vi "氨氮总磷质控流程.vi"(0 "队列输入":refnum<queue>, 5 "氨氮":bool, 7 "氨氮量程切换":enum32{"H", "L", "AUTO"}(ring)=enum."AUTO", 9 "总磷":bool, 11 "总磷量程切换":enum32{"H", "L", "AUTO"}(ring)=enum."AUTO") -> (4 "布尔":bool, 6 "总磷中断报警":bool, 8 "氨氮中断报警":bool)   [LabVIEW 2016, in "质控单元.lvlib"]
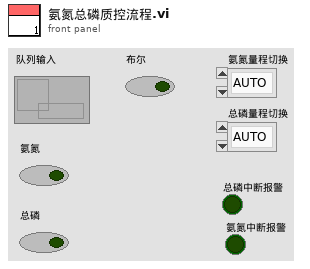
[diagram p1: front panel]
types:
  T1 = enum16{"待机", "启动氨氮水样", "氨氮测量中", "启动氨氮加标", "启动氨氮加标回收", "氨氮加标回收测量中", "启动总磷水样", "总磷水样测量中", "启动总磷加标", "启动总磷加标回收", "总磷加标回收测量中", "结束"}
  T2 = cluster{"站号":u16, "量程切换":enum32{"H", "L", "AUTO"}, "控制命令":enum16{"启动测量", "标样核查", "零点核查", "跨度核查", "空白测试", "平行样测试", "加标回收", "空白校准", "标样校准", "初始化（清洗）", "停止测试", "仪器重启", "校时", "模式设置", "测量间隔设置", "盲样测试"}, "模式设置":enum16{"待机", "连续模式", "周期模式", "定点模式", "受控模式", "手动模式"}, "测量间隔":u16}
  T3 = cluster{"时间标识":timestamp, "设备":string, "日志信息":string}
  T4 = cluster{"系统时间":timestamp, "工作状态":enum16{"空闲", "水样测试", "标样核查", "零点核查", "跨度核查", "空白测试", "平行样测试", "加标回收", "空白校准", "标样校准", "初始化（清洗）"}, "测量模式":enum16{"待机", "连续模式", "周期模式", "定点模式", "受控模式", "手动模式"}, "告警代码":enum16{"无告警", "缺试剂告警", "缺水样告警", "缺蒸馏水告警", "缺标液告警", "仪表漏液告警", "标定异常告警", "超量程告警", "加热异常", "低试剂预警", "超上限告警", "超下限告警", "仪表内部其他异常", "滴定异常告警", "电极异常告警", "量程切换告警", "参数设置告警", "PH电极电位异常", "电导率电极异常", "浊度光度异常", "溶解氧电极异常", "溶解氧光强异常", "温度异常告警", "PH异常告警", "溶解氧异常告警", "电导率异常告警", "浊度异常告警", "叶绿素异常告警", "藻密度异常告警", "蓝绿藻异常告警", "ORP异常告警", "氨氮异常告警", "清洁刷异常告警", "SD卡异常告警", "蓝牙异常告警", "Wifi异常告警", "流程异常告警"}, "故障代码":enum16{"无故障", "电机故障", "温度故障", "通讯故障", "滴定故障"}, "日志代码":u16, "软件版本":u16, "F0":sgl, "F1":sgl, "F2":sgl, "F3":sgl, "T":sgl, "H":sgl, "id":u16, "flowid":u16, "量程":u16, "总磷控温温度1":sgl, "营养盐控温温度2":sgl, "ADC":sgl}
  T5 = enum16{"空闲", "水样测试", "标样核查", "零点核查", "跨度核查", "空白测试", "平行样测试", "加标回收", "空白校准", "标样校准", "初始化（清洗）"}
  T6 = cluster{"因子编码":u32, "单位":u16, "标样参考值":sgl, "水样数据时间":timestamp, "水样实测值":sgl, "水样数据标识":string, "标样数据时间":timestamp, "标样实测值":sgl, "标样数据标识":string, "空白数据时间":timestamp, "空白实测值":sgl, "空白数据标识":string, "零点核查数据时间":timestamp, "零点核查实测值":sgl, "零点核查数据标识":string, "跨度核查数据时间":timestamp, "跨度核查实测值":sgl, "跨度核查数据标识":string, "加标回收数据时间":timestamp, "加标回收实测值":sgl, "加标回收数据标识":string, "平行样数据时间":timestamp, "平行样实测值":sgl, "平行样数据标识":string}
  T7 = cluster{"量程":dbl, "检出限":dbl, "加标前水样浓度":dbl, "加标后水样浓度":dbl, "加标水杯定容体积":dbl, "加标母液浓度":dbl, "加标体积":dbl, "加标回收率":dbl}
  T8 = cluster{"氨氮":u8, "总磷":u8, "总氮":u8, "CODMn":u8, "CODCr":u8}
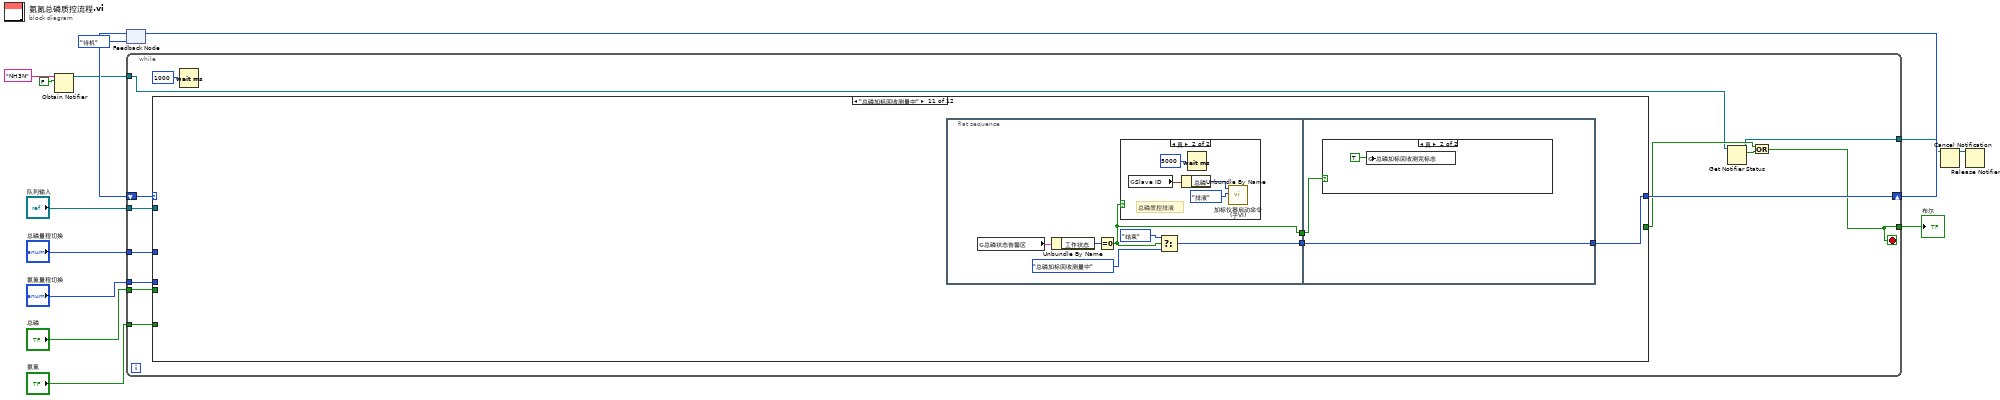
[diagram p0: block diagram]
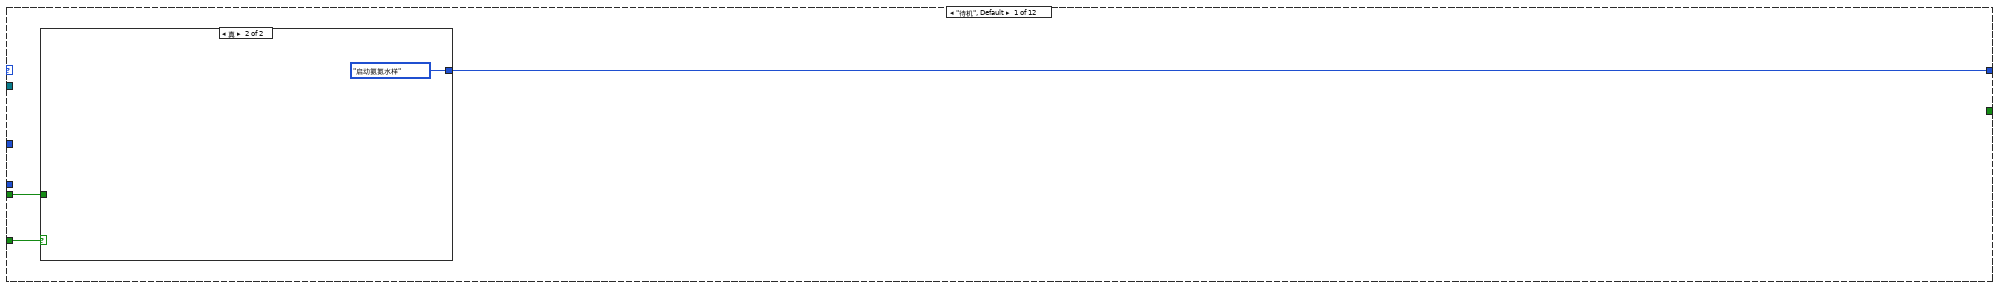
[diagram p2: hidden frame]
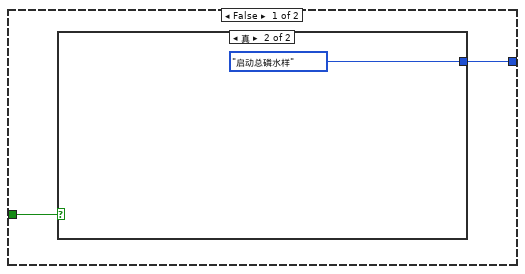
[diagram p3: hidden frame]
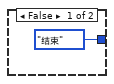
[diagram p4: hidden frame]
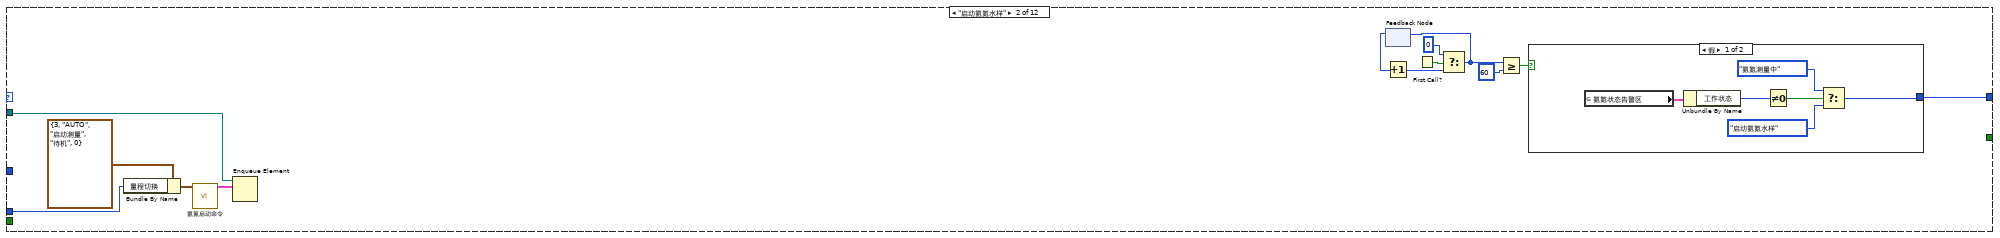
[diagram p5: hidden frame]
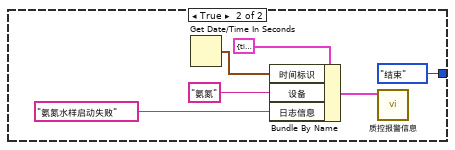
[diagram p6: hidden frame]
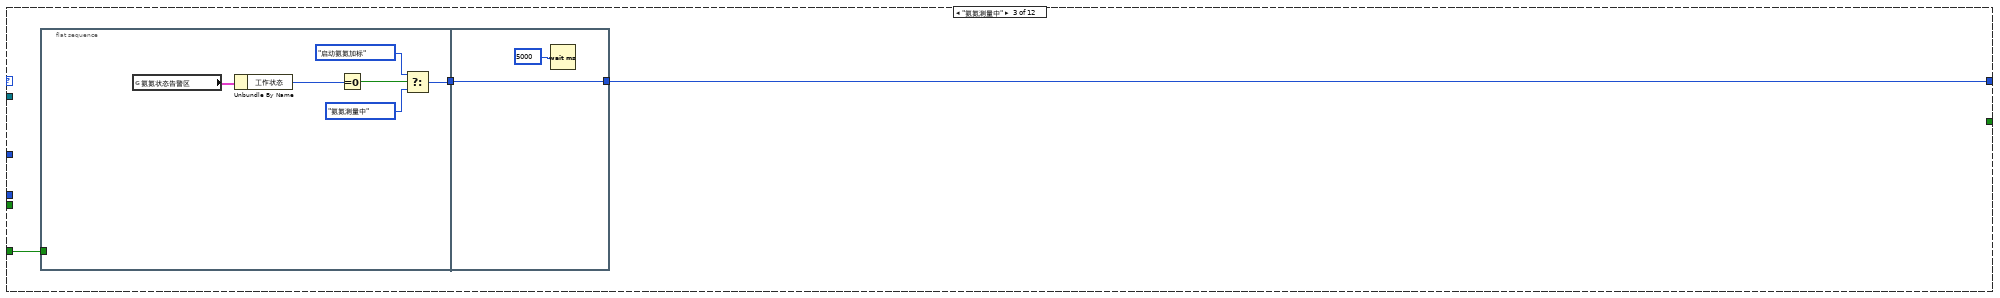
[diagram p7: hidden frame]
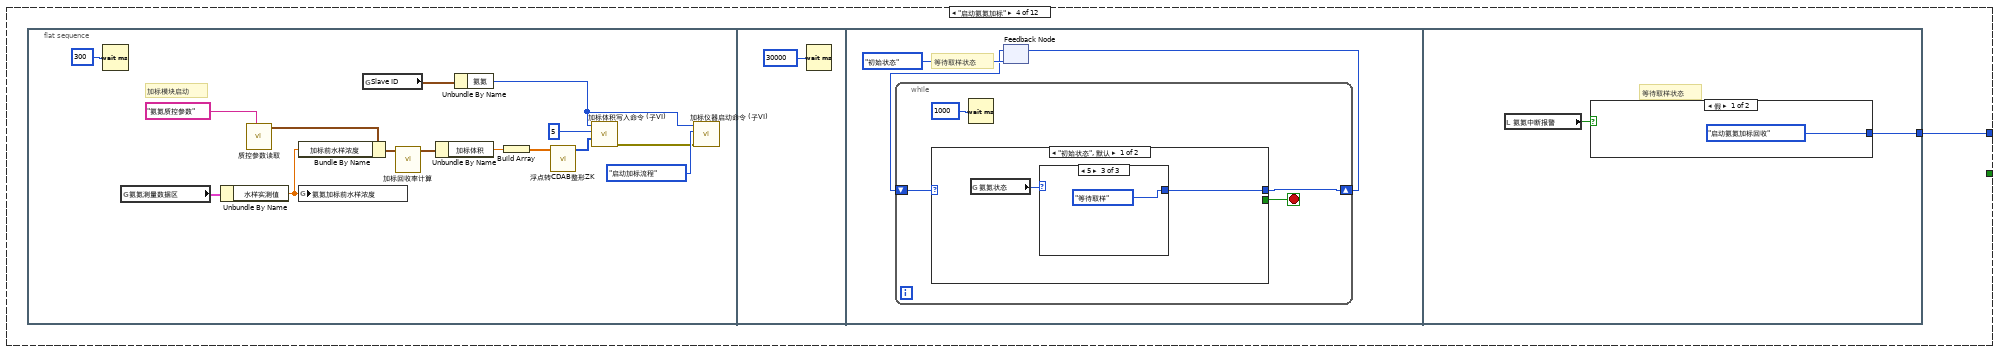
[diagram p8: hidden frame]
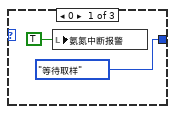
[diagram p9: hidden frame]
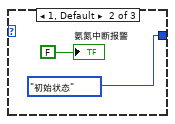
[diagram p10: hidden frame]
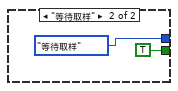
[diagram p11: hidden frame]
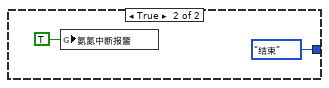
[diagram p12: hidden frame]
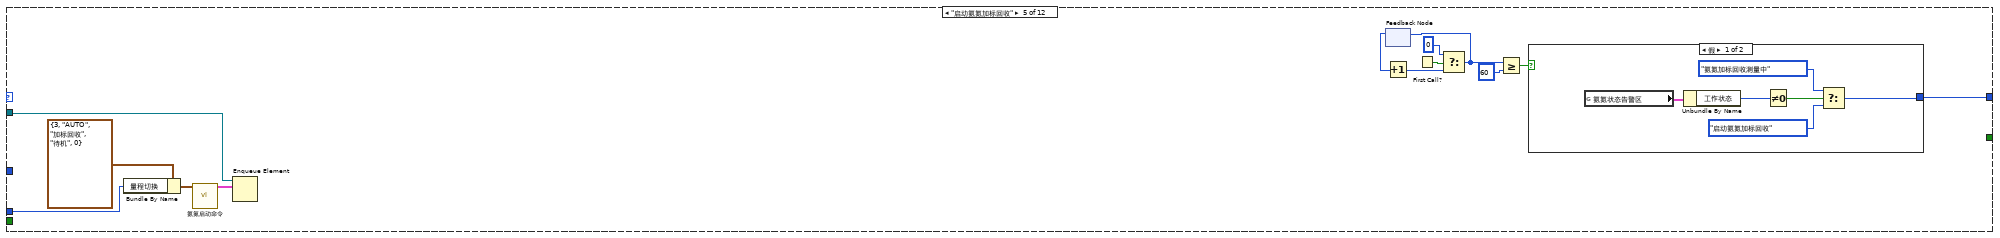
[diagram p13: hidden frame]
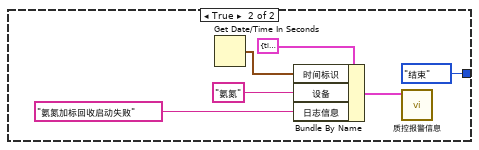
[diagram p14: hidden frame]
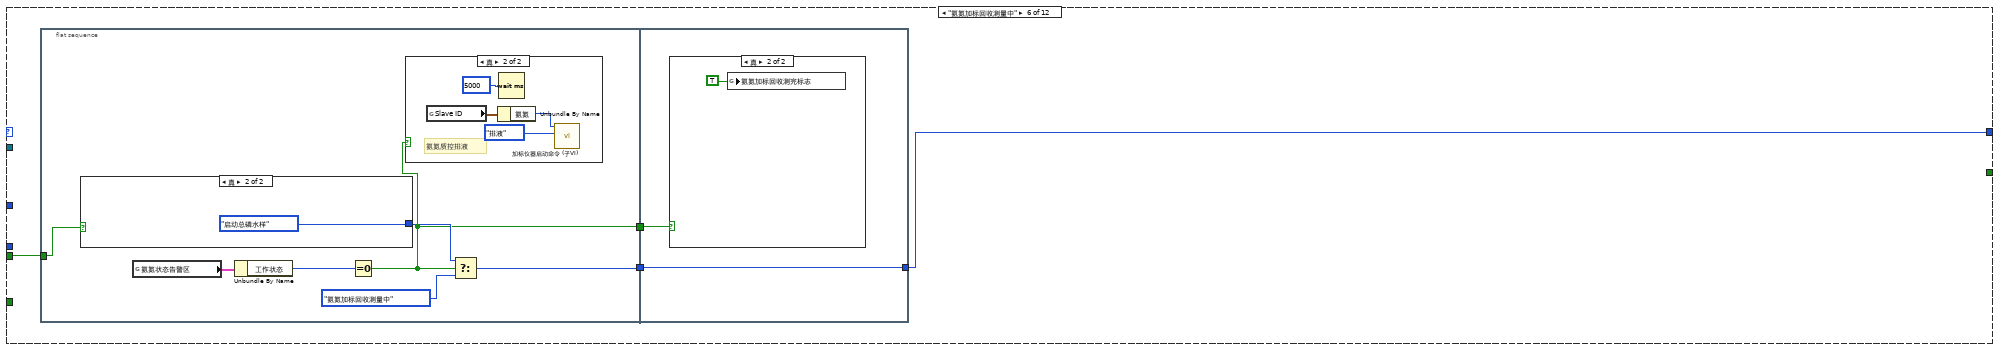
[diagram p15: hidden frame]
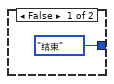
[diagram p16: hidden frame]
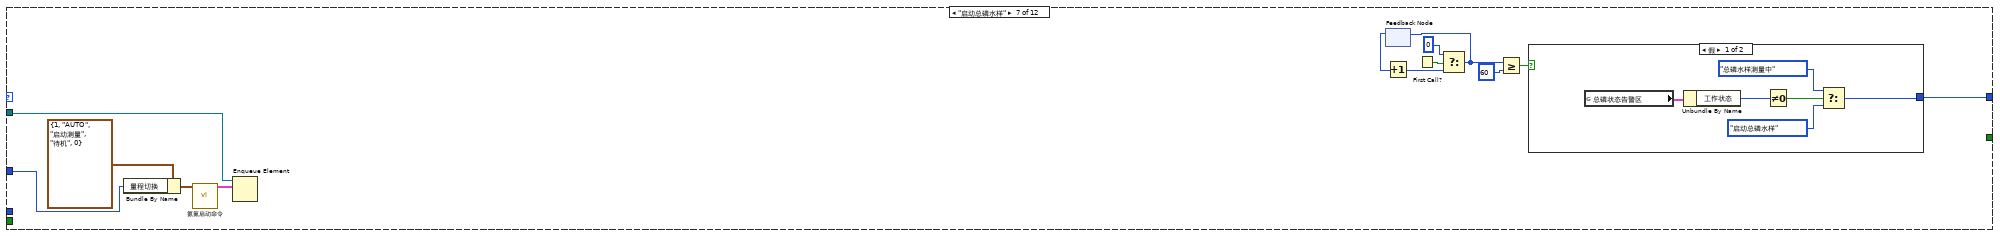
[diagram p19: hidden frame]
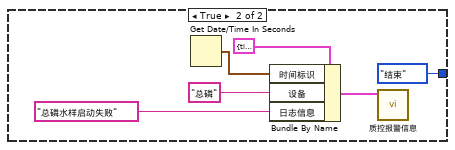
[diagram p20: hidden frame]
diagram:
  n1 = Obtain Notifier(name (unnamed)="NH3N" ("名称（未命名）"), notification data type=FALSE) -> (notifier out=w3:refnum<notifier>)  [unwired: 2 in, 2 out]
  n2 = feedback #1(T1."待机") -> (w13:T1)
  n3 = while {
    tunnel: "总磷" -> [w25]
    tunnel: "队列输入" -> [w24]
    tunnel: "氨氮量程切换" -> [w23]
    tunnel: "总磷量程切换" -> [w22]
    tunnel: "氨氮" -> [w21]
    tunnel: [w17] -> w6
    shift-right: [w26] -> w12
    shift-left: w13 -> [w27]
    tunnel: w3 -> [w16]
    tunnel: [w15] -> w1
    stop <- w17 stop-if-true
    n4 = case shown="\"总磷加标回收测量中\"" w27 {
      tunnel: [w30 w47 w63 w72 w114 w137 w166 w182 w191 w233 w255 T1."结束"] -> w26
      tunnel: w24 -> [_ w48 _ _ w115 _ w167 _ _ w234 _ _]
      tunnel: [_ _ _ _ _ _ _ _ _ _ _ TRUE] -> w18
      tunnel: w25 -> [w28 _ _ _ _ w136 _ w180 _ _ _ _]
      tunnel: w21 -> [w29 _ w61 _ _ _ _ _ _ _ _ _]
      tunnel: w23 -> [_ w37 _ _ w111 _ _ _ _ _ _ _]
      tunnel: w22 -> [_ _ _ _ _ _ w155 _ _ w232 _ _]
      frame "待机", Default {
        n5 = case shown="真" w29 {
          tunnel: [w31 T1."启动氨氮水样"] -> w30
          tunnel: w28 -> [w32 _]
          frame False {
            n6 = case shown="真" w32 {
              tunnel: [T1."结束" T1."启动总磷水样"] -> w31
              frame False {
              }
              frame True {
              }
            }
          }
          frame True {
          }
        }
      }
      frame "启动氨氮水样" {
        n7 = Bundle By Name(cluster=T2 {"站号"=3, "量程切换"=enum."AUTO", "控制命令"=enum."启动测量", "模式设置"=enum."待机", "测量间隔"=0} ("参数"), "量程切换"=w37) -> (w36:T2)
        n8 = call "氨氮启动命令.vi"("参数"=w36) -> ("启动命令"=w39:cluster{"命令":string, "data":variant})  [unwired: 10 in]
        n9 = Enqueue Element(queue=w48, element=w39) -> ()  [unwired: 2 in, 3 out]
        n10 = feedback #2() -> (w44:i32)  [unwired: 1 in]
        n11 = Increment(x=w44) -> (x+1=w43:i32)
        n12 = First Call?() -> (First Call?: T/F=w45:bool)
        n13 = Select(t=0, s=w45, f=w43) -> (s? t:f=w42:i32)
        n14 = feedback-in #2(w42) -> ()
        n15 = Greater Or Equal?(x=w42, y=60) -> (x >= y?=w40:bool)
        n16 = case shown="假" w40 {
          tunnel: [w52 T1."结束"] -> w47
          frame False {
            n17 = global read "与氨氮交互全局.vi" "氨氮状态告警区"() -> (w49:T4)
            n18 = Unbundle By Name(w49) -> ("工作状态"=w54:T5)
            n19 = Not Equal To 0?(x=w54) -> (x != 0?=w53:bool)
            n20 = Select(t=T1."氨氮测量中", s=w53, f=T1."启动氨氮水样") -> (s? t:f=w52:T1)
          }
          frame True {
            n21 = Get Date/Time In Seconds() -> (seconds since 1Jan1904=w60:timestamp)
            n22 = Bundle By Name(cluster=T3 {"时间标识"=timestamp(0 s since 1904-01-01), "设备"="", "日志信息"=""} ("data in"), "时间标识"=w60, "设备"="氨氮", "日志信息"="氨氮水样启动失败") -> (w56:T3)
            n23 = call "质控报警信息.vi"("data in"=w56) -> ()  [unwired: 10 in, 1 out]
          }
        }
      }
      frame "氨氮测量中" {
        n24 = flat-sequence {
          tunnel: [w68] -> w62
          tunnel: w61 -> [_]
          tunnel: [w71] -> w63
          tunnel: w62 -> [w71]
          frame #0 {
            n25 = global read "与氨氮交互全局.vi" "氨氮状态告警区"() -> (w64:T4)
            n26 = Unbundle By Name(w64) -> ("工作状态"=w69:T5)
            n27 = Equal To 0?(x=w69) -> (x = 0?=w67:bool)
            n28 = Select(t=T1."启动氨氮加标", s=w67, f=T1."氨氮测量中") -> (s? t:f=w68:T1)
          }
          frame #1 {
            n29 = Wait (ms)(milliseconds to wait=u32 5000 ("等待时间（毫秒）")) -> ()  [unwired: 1 out]
          }
        }
      }
      frame "启动氨氮加标" {
        n30 = flat-sequence {
          tunnel: [w106] -> w72
          frame #0 {
            # "加标模块启动"
            n31 = Wait (ms)(milliseconds to wait=u32 300 ("等待时间（毫秒）")) -> ()  [unwired: 1 out]
            n32 = global read "与氨氮交互全局.vi" "氨氮测量数据区"() -> (w80:T6)
            n33 = Unbundle By Name(w80) -> ("水样实测值"=w81:sgl)
            n34 = call "质控参数读取.vi"("section"="氨氮质控参数") -> ("参数"=w85:T7)  [unwired: 9 in, 1 out]
            n35 = Bundle By Name(cluster=w85, "加标前水样浓度"=w81) -> (w86:T7)
            n36 = global write "水样浓度全局.vi" "氨氮加标前水样浓度"(w81) -> ()
            n37 = global read "断电保存全局.vi" "Slave ID"() -> (w78:T8)
            n38 = call "加标回收率计算.vi"("参数"=w86) -> ("参数 out"=w84:T7)  [unwired: 9 in, 1 out]
            n39 = Unbundle By Name(w84) -> ("加标体积"=w82:dbl)
            n40 = Unbundle By Name(w78) -> ("氨氮"=w73:u8)
            n41 = Build Array(w82) -> (w83:dbl[])
            n42 = call "浮点转CDAB整形ZK.vi"("浮点数"=w83) -> ("CDAB整形输出"=w74:u16[])  [unwired: 10 in]
            n43 = call "加标体积写入命令 (子VI).vi"("values"=w74, "starting address"=u16 5, "Slave ID"=w73) -> ("错误输出"=w76:errorcluster)  [unwired: 8 in]
            n44 = call "加标仪器启动命令 (子VI).vi"("错误输入（无错误）"=w76, "启动命令"=enum16{"启动水样流程", "启动加标流程", "排液", "停止"}."启动加标流程", "仪器"=w73) -> ()  [unwired: 8 in, 1 out]
          }
          frame #1 {
            n45 = Wait (ms)(milliseconds to wait=u32 30000 ("等待时间（毫秒）")) -> ()  [unwired: 1 out]
          }
          frame #2 {
            # "等待取样状态"
            n46 = feedback #3(enum16{"初始状态", "等待取样"}."初始状态") -> (w90:enum16{"初始状态", "等待取样"})
            n47 = while {
              shift-right: [w94] -> w89
              shift-left: w90 -> [w95]
              stop <- w93 stop-if-true
              n48 = case shown="\"初始状态\", 默认" w95 {
                tunnel: [w97 enum16{"初始状态", "等待取样"}."等待取样"] -> w94
                tunnel: [_ TRUE] -> w93
                frame "初始状态", Default {
                  n49 = global read "加标回收状态全局变量.vi" "氨氮状态"() -> (w96:u16)
                  n50 = case shown="5" w96 {
                    tunnel: [enum16{"初始状态", "等待取样"}."等待取样" enum16{"初始状态", "等待取样"}."初始状态" enum16{"初始状态", "等待取样"}."等待取样"] -> w97
                    frame 0 {
                      n51 = local write "氨氮中断报警"(TRUE ("氨氮中断报警")) -> ()
                    }
                    frame 1, Default {
                      "氨氮中断报警" <- FALSE ("氨氮中断报警")
                    }
                    frame 5 {
                    }
                  }
                }
                frame "等待取样" {
                }
              }
              n52 = Wait (ms)(milliseconds to wait=u32 1000 ("等待时间（毫秒）")) -> ()  [unwired: 1 out]
            }
            n53 = feedback-in #3(w89) -> ()
          }
          frame #3 {
            # "等待取样状态"
            n54 = local read "氨氮中断报警"() -> (w105:bool)
            n55 = case shown="假" w105 {
              tunnel: [T1."启动氨氮加标回收" T1."结束"] -> w106
              frame False {
              }
              frame True {
                n56 = global write "质控中断报警全局.vi" "氨氮中断报警"(TRUE ("氨氮中断报警")) -> ()
              }
            }
          }
        }
      }
      frame "启动氨氮加标回收" {
        n57 = Bundle By Name(cluster=T2 {"站号"=3, "量程切换"=enum."AUTO", "控制命令"=enum."加标回收", "模式设置"=enum."待机", "测量间隔"=0} ("参数"), "量程切换"=w111) -> (w110:T2)
        n58 = call "氨氮启动命令.vi"("参数"=w110) -> ("启动命令"=w113:cluster{"命令":string, "data":variant})  [unwired: 10 in]
        n59 = Enqueue Element(queue=w115, element=w113) -> ()  [unwired: 2 in, 3 out]
        n60 = feedback #4() -> (w120:i32)  [unwired: 1 in]
        n61 = Increment(x=w120) -> (x+1=w119:i32)
        n62 = First Call?() -> (First Call?: T/F=w121:bool)
        n63 = Select(t=0, s=w121, f=w119) -> (s? t:f=w118:i32)
        n64 = feedback-in #4(w118) -> ()
        n65 = Greater Or Equal?(x=w118, y=60) -> (x >= y?=w116:bool)
        n66 = case shown="假" w116 {
          tunnel: [w126 T1."结束"] -> w114
          frame False {
            n67 = global read "与氨氮交互全局.vi" "氨氮状态告警区"() -> (w123:T4)
            n68 = Unbundle By Name(w123) -> ("工作状态"=w128:T5)
            n69 = Not Equal To 0?(x=w128) -> (x != 0?=w127:bool)
            n70 = Select(t=T1."氨氮加标回收测量中", s=w127, f=T1."启动氨氮加标回收") -> (s? t:f=w126:T1)
          }
          frame True {
            n71 = Get Date/Time In Seconds() -> (seconds since 1Jan1904=w134:timestamp)
            n72 = Bundle By Name(cluster=T3 {"时间标识"=timestamp(0 s since 1904-01-01), "设备"="", "日志信息"=""} ("data in"), "时间标识"=w134, "设备"="氨氮", "日志信息"="氨氮加标回收启动失败") -> (w130:T3)
            n73 = call "质控报警信息.vi"("data in"=w130) -> ()  [unwired: 10 in, 1 out]
          }
        }
      }
      frame "氨氮加标回收测量中" {
        n74 = flat-sequence {
          tunnel: [w144] -> w138
          tunnel: w136 -> [w141]
          tunnel: [w139] -> w135
          tunnel: [w153] -> w137
          tunnel: w138 -> [w153]
          tunnel: w135 -> [w152]
          frame #0 {
            n75 = case shown="真" w141 {
              tunnel: [T1."结束" T1."启动总磷水样"] -> w142
              frame False {
              }
              frame True {
              }
            }
            n76 = global read "与氨氮交互全局.vi" "氨氮状态告警区"() -> (w140:T4)
            n77 = Unbundle By Name(w140) -> ("工作状态"=w145:T5)
            n78 = Equal To 0?(x=w145) -> (x = 0?=w139:bool)
            n79 = case shown="真" w139 {
              frame False {
              }
              frame True {
                # "氨氮质控排液"
                n80 = global read "断电保存全局.vi" "Slave ID"() -> (w149:T8)
                n81 = Unbundle By Name(w149) -> ("氨氮"=w148:u8)
                n82 = Wait (ms)(milliseconds to wait=u32 5000 ("等待时间（毫秒）")) -> ()  [unwired: 1 out]
                n83 = call "加标仪器启动命令 (子VI).vi"("启动命令"=enum16{"启动水样流程", "启动加标流程", "排液", "停止"}."排液", "仪器"=w148) -> ()  [unwired: 9 in, 1 out]
              }
            }
            n84 = Select(t=w142, s=w139, f=T1."氨氮加标回收测量中") -> (s? t:f=w144:T1)
          }
          frame #1 {
            n85 = case shown="真" w152 {
              frame False {
              }
              frame True {
                n86 = global write "质控测完标志全局 1.vi" "氨氮加标回收测完标志"(TRUE) -> ()
              }
            }
          }
        }
      }
      frame "启动总磷水样" {
        n87 = Bundle By Name(cluster=T2 {"站号"=1, "量程切换"=enum."AUTO", "控制命令"=enum."启动测量", "模式设置"=enum."待机", "测量间隔"=0} ("参数"), "量程切换"=w155) -> (w157:T2)
        n88 = call "氨氮启动命令.vi"("参数"=w157) -> ("启动命令"=w156:cluster{"命令":string, "data":variant})  [unwired: 10 in]
        n89 = Enqueue Element(queue=w167, element=w156) -> ()  [unwired: 2 in, 3 out]
        n90 = feedback #5() -> (w163:i32)  [unwired: 1 in]
        n91 = Increment(x=w163) -> (x+1=w162:i32)
        n92 = First Call?() -> (First Call?: T/F=w164:bool)
        n93 = Select(t=0, s=w164, f=w162) -> (s? t:f=w161:i32)
        n94 = feedback-in #5(w161) -> ()
        n95 = Greater Or Equal?(x=w161, y=60) -> (x >= y?=w159:bool)
        n96 = case shown="假" w159 {
          tunnel: [w171 T1."结束"] -> w166
          frame False {
            n97 = global read "与总磷交互全局.vi" "总磷状态告警区"() -> (w168:T4)
            n98 = Unbundle By Name(w168) -> ("工作状态"=w172:T5)
            n99 = Not Equal To 0?(x=w172) -> (x != 0?=w173:bool)
            n100 = Select(t=T1."总磷水样测量中", s=w173, f=T1."启动总磷水样") -> (s? t:f=w171:T1)
          }
          frame True {
            n101 = Get Date/Time In Seconds() -> (seconds since 1Jan1904=w179:timestamp)
            n102 = Bundle By Name(cluster=T3 {"时间标识"=timestamp(0 s since 1904-01-01), "设备"="", "日志信息"=""} ("data in"), "时间标识"=w179, "设备"="总磷", "日志信息"="总磷水样启动失败") -> (w175:T3)
            n103 = call "质控报警信息.vi"("data in"=w175) -> ()  [unwired: 10 in, 1 out]
          }
        }
      }
      frame "总磷水样测量中" {
        n104 = flat-sequence {
          tunnel: [w187] -> w181
          tunnel: w180 -> [_]
          tunnel: [w190] -> w182
          tunnel: w181 -> [w190]
          frame #0 {
            n105 = global read "与总磷交互全局.vi" "总磷状态告警区"() -> (w183:T4)
            n106 = Unbundle By Name(w183) -> ("工作状态"=w188:T5)
            n107 = Equal To 0?(x=w188) -> (x = 0?=w186:bool)
            n108 = Select(t=T1."启动总磷加标", s=w186, f=T1."总磷水样测量中") -> (s? t:f=w187:T1)
          }
          frame #1 {
            n109 = Wait (ms)(milliseconds to wait=u32 5000 ("等待时间（毫秒）")) -> ()  [unwired: 1 out]
          }
        }
      }
      frame "启动总磷加标" {
        n110 = flat-sequence {
          tunnel: [w225] -> w191
          frame #0 {
            # "加标模块启动"
            n111 = global read "与总磷交互全局.vi" "总磷测量数据区"() -> (w198:T6)
            n112 = Wait (ms)(milliseconds to wait=u32 300 ("等待时间（毫秒）")) -> ()  [unwired: 1 out]
            n113 = Unbundle By Name(w198) -> ("水样实测值"=w200:sgl)
            n114 = call "质控参数读取.vi"("section"="总磷质控参数") -> ("参数"=w201:T7)  [unwired: 9 in, 1 out]
            n115 = Bundle By Name(cluster=w201, "加标前水样浓度"=w200) -> (w205:T7)
            n116 = global write "水样浓度全局.vi" "总磷加标前水样浓度"(w200) -> ()
            n117 = call "加标回收率计算.vi"("参数"=w205) -> ("参数 out"=w204:T7)  [unwired: 9 in, 1 out]
            n118 = global read "断电保存全局.vi" "Slave ID"() -> (w193:T8)
            n119 = Unbundle By Name(w204) -> ("加标体积"=w202:dbl)
            n120 = Unbundle By Name(w193) -> ("总磷"=w192:u8)
            n121 = Build Array(w202) -> (w203:dbl[])
            n122 = call "浮点转CDAB整形ZK.vi"("浮点数"=w203) -> ("CDAB整形输出"=w194:u16[])  [unwired: 10 in]
            n123 = call "加标体积写入命令 (子VI).vi"("values"=w194, "starting address"=u16 5, "Slave ID"=w192) -> ("错误输出"=w196:errorcluster)  [unwired: 8 in]
            n124 = call "加标仪器启动命令 (子VI).vi"("错误输入（无错误）"=w196, "启动命令"=enum16{"启动水样流程", "启动加标流程", "排液", "停止"}."启动加标流程", "仪器"=w192) -> ()  [unwired: 8 in, 1 out]
          }
          frame #1 {
            n125 = Wait (ms)(milliseconds to wait=u32 30000 ("等待时间（毫秒）")) -> ()  [unwired: 1 out]
          }
          frame #2 {
            # "等待取样状态"
            n126 = feedback #6(enum16{"初始状态", "等待取样"}."初始状态") -> (w210:enum16{"初始状态", "等待取样"})
            n127 = while {
              shift-right: [w213] -> w209
              shift-left: w210 -> [w214]
              stop <- w212 stop-if-true
              n128 = case shown="\"初始状态\", 默认" w214 {
                tunnel: [w216 enum16{"初始状态", "等待取样"}."等待取样"] -> w213
                tunnel: [_ TRUE] -> w212
                frame "初始状态", Default {
                  n129 = global read "加标回收状态全局变量.vi" "总磷状态"() -> (w215:u16)
                  n130 = case shown="5" w215 {
                    tunnel: [enum16{"初始状态", "等待取样"}."等待取样" enum16{"初始状态", "等待取样"}."初始状态" enum16{"初始状态", "等待取样"}."等待取样"] -> w216
                    frame 0 {
                      n131 = local write "总磷中断报警"(TRUE ("总磷中断报警")) -> ()
                    }
                    frame 1, Default {
                      "总磷中断报警" <- FALSE ("总磷中断报警")
                    }
                    frame 5 {
                    }
                  }
                }
                frame "等待取样" {
                }
              }
              n132 = Wait (ms)(milliseconds to wait=u32 1000 ("等待时间（毫秒）")) -> ()  [unwired: 1 out]
            }
            n133 = feedback-in #6(w209) -> ()
          }
          frame #3 {
            # "等待取样状态"
            n134 = local read "总磷中断报警"() -> (w224:bool)
            n135 = case shown="真" w224 {
              tunnel: [T1."启动总磷加标回收" T1."结束"] -> w225
              frame False {
              }
              frame True {
                n136 = global write "质控中断报警全局.vi" "总磷中断报警"(TRUE ("总磷中断报警")) -> ()
              }
            }
          }
        }
      }
      frame "启动总磷加标回收" {
        n137 = Bundle By Name(cluster=T2 {"站号"=1, "量程切换"=enum."AUTO", "控制命令"=enum."加标回收", "模式设置"=enum."待机", "测量间隔"=0} ("参数"), "量程切换"=w232) -> (w230:T2)
        n138 = call "氨氮启动命令.vi"("参数"=w230) -> ("启动命令"=w229:cluster{"命令":string, "data":variant})  [unwired: 10 in]
        n139 = Enqueue Element(queue=w234, element=w229) -> ()  [unwired: 2 in, 3 out]
        n140 = feedback #7() -> (w239:i32)  [unwired: 1 in]
        n141 = Increment(x=w239) -> (x+1=w238:i32)
        n142 = First Call?() -> (First Call?: T/F=w240:bool)
        n143 = Select(t=0, s=w240, f=w238) -> (s? t:f=w237:i32)
        n144 = feedback-in #7(w237) -> ()
        n145 = Greater Or Equal?(x=w237, y=60) -> (x >= y?=w235:bool)
        n146 = case shown="假" w235 {
          tunnel: [w246 T1."结束"] -> w233
          frame False {
            n147 = global read "与总磷交互全局.vi" "总磷状态告警区"() -> (w243:T4)
            n148 = Unbundle By Name(w243) -> ("工作状态"=w242:T5)
            n149 = Not Equal To 0?(x=w242) -> (x != 0?=w247:bool)
            n150 = Select(t=T1."总磷加标回收测量中", s=w247, f=T1."启动总磷加标回收") -> (s? t:f=w246:T1)
          }
          frame True {
            n151 = Get Date/Time In Seconds() -> (seconds since 1Jan1904=w253:timestamp)
            n152 = Bundle By Name(cluster=T3 {"时间标识"=timestamp(0 s since 1904-01-01), "设备"="", "日志信息"=""} ("data in"), "时间标识"=w253, "设备"="总磷", "日志信息"="总磷启动失败") -> (w249:T3)
            n153 = call "质控报警信息.vi"("data in"=w249) -> ()  [unwired: 10 in, 1 out]
          }
        }
      }
      frame "总磷加标回收测量中" {
        n154 = flat-sequence {
          tunnel: [w262] -> w256
          tunnel: [w257] -> w254
          tunnel: [w268] -> w255
          tunnel: w256 -> [w268]
          tunnel: w254 -> [w267]
          frame #0 {
            n155 = global read "与总磷交互全局.vi" "总磷状态告警区"() -> (w259:T4)
            n156 = Unbundle By Name(w259) -> ("工作状态"=w258:T5)
            n157 = Equal To 0?(x=w258) -> (x = 0?=w257:bool)
            n158 = case shown="真" w257 {
              frame False {
              }
              frame True {
                # "总磷质控排液"
                n159 = global read "断电保存全局.vi" "Slave ID"() -> (w264:T8)
                n160 = Unbundle By Name(w264) -> ("总磷"=w265:u8)
                n161 = Wait (ms)(milliseconds to wait=u32 5000 ("等待时间（毫秒）")) -> ()  [unwired: 1 out]
                n162 = call "加标仪器启动命令 (子VI).vi"("启动命令"=enum16{"启动水样流程", "启动加标流程", "排液", "停止"}."排液", "仪器"=w265) -> ()  [unwired: 9 in, 1 out]
              }
            }
            n163 = Select(t=T1."结束", s=w257, f=T1."总磷加标回收测量中") -> (s? t:f=w262:T1)
          }
          frame #1 {
            n164 = case shown="真" w267 {
              frame False {
              }
              frame True {
                n165 = global write "质控测完标志全局 1.vi" "总磷加标回收测完标志"(TRUE) -> ()
              }
            }
          }
        }
      }
      frame "结束" {
        n166 = Wait (ms)(milliseconds to wait=u32 5000 ("等待时间（毫秒）")) -> ()  [unwired: 1 out]
      }
    }
    n167 = Wait (ms)(milliseconds to wait=u32 1000 ("等待时间（毫秒）")) -> ()  [unwired: 1 out]
    n168 = Get Notifier Status(notifier=w16) -> (notifier out=w15:refnum<notifier>, current notification=w19:bool)  [unwired: 1 in, 3 out]
    n169 = Or(x=w18, y=w19) -> (x .or. y?=w17:bool)
  }
  "布尔" <- w6
  n170 = feedback-in #1(w12) -> ()
  n171 = Cancel Notification(0:w1) -> (8:w2:refnum<notifier>)  [unwired: 1 in, 2 out]
  n172 = Release Notifier(notifier=w2) -> ()  [unwired: 2 in, 3 out]
